vi "Build New Ballard MIL-STD-1553 Custom Device.vi"() -> ()   [LabVIEW 2020]
uses:
  <vilib>/addons/VeriStand Custom Device Scripting APIs/Ballard MIL-STD-1553/Shared/Address.ctl
  <vilib>/addons/VeriStand Custom Device Scripting APIs/Ballard MIL-STD-1553/Shared/Device Parameters.ctl
  <vilib>/addons/VeriStand Custom Device Scripting APIs/Ballard MIL-STD-1553/Shared/Initialization Method.ctl
  NationalInstruments.VeriStand.SystemDefinitionAPI
  AIM MIL-STD-1553 Scripting Example Support.lvlib
panel:
  in  "Example Documentation":string="Overview: Demonstrates using the Ballard MIL-STD-1553 scripting API to add and configure a new custom device from configuration data. \n\nInstructions:\n1. Specify the PXI Slot Number and Core Number for your Astronics MIL-STD-1553 hardware with Ballard technology.\n2. Specify the Hardware Configuration File. The hardware configuration file must be consistent with the schema installed by the Ballard hardware driver at \nC:\\Program Files (x86)\\Astronics Ballard Technology LabVIEW Driver\\Help\\index.html.\n3. (VeriStand) Optionally, to perform avionics bus communications with Ballard MIL-STD-1553 hardware you may:\n   a. Open the Ballard MIL-STD-1553 System Definition in VeriStand.\n   b. Configure the PXI Linux RT Target.\n   c. Deploy the scripted system definition."
  in  "Core Number":i32
  in  "PXI Slot Number":i32=2
  in  "Hardware Configuration File":path=path "Support/Ballard MIL-STD-1553 Hardware.xml"
  in  "Base System Definition File":path=path "Support/Base.nivssdf"
  in  "Output System Definition File":path=path "Support/Scripted Configuration Ballard MIL-STD-1553.nivssdf"
  out "Ballard MIL-STD-1553 System Definition":path
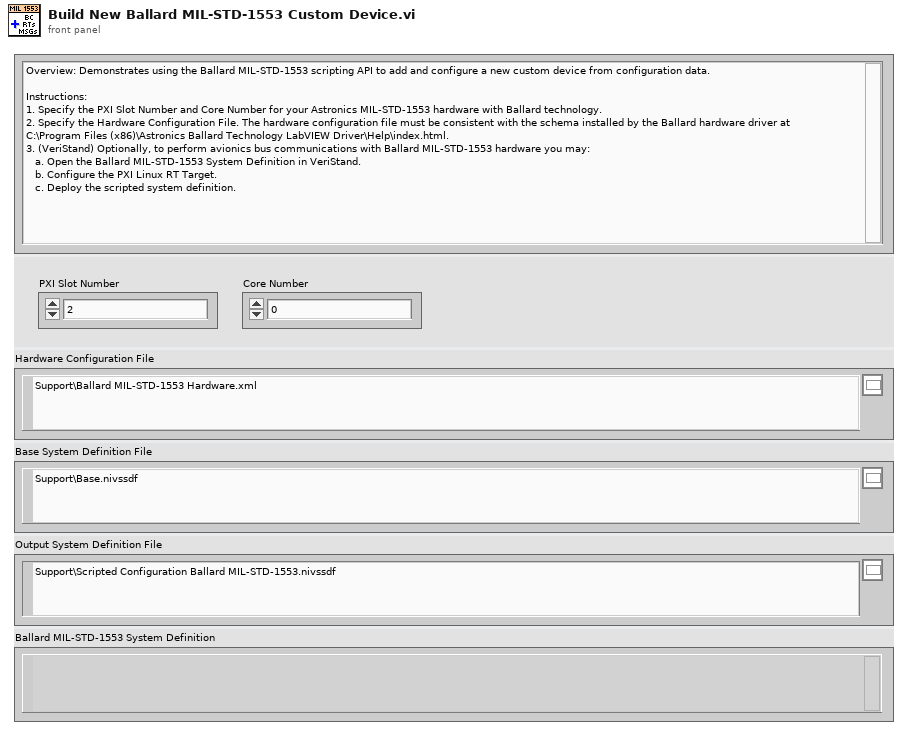
[diagram p1: front panel]
types:
  T1 = typedef "Device Parameters.ctl" = cluster{"initialization method":T2, "card number":i32, "PXI slot number":i32, "core number":i32}
  T2 = typedef "Initialization Method.ctl" = enum16{"PXI Slot Number", "Card Number"}
  T3 = typedef "Address.ctl" = u16
  T4 = cluster{"name":string, "message type":string, "Tx endpoint":cluster{"terminal address":u16, "subaddress":u16}, "Rx endpoint":cluster{"terminal address":u16, "subaddress":u16}, "create timestamp ch":bool, "mode code":u16, "number of words":u16, "parameters":cluster{"name":string, "default value":dbl, "unit":string, "parameter definition":cluster{"start index":i32, "size (bits)":i32, "encoding":enum16{"BNR", "BCD", "Discrete"}, "signed":bool, "multiplier":dbl, "offset":dbl}}[]}[]
  T5 = typedef "Custom Device API.lvlib/Custom Device Item Ref.ctl" = u64
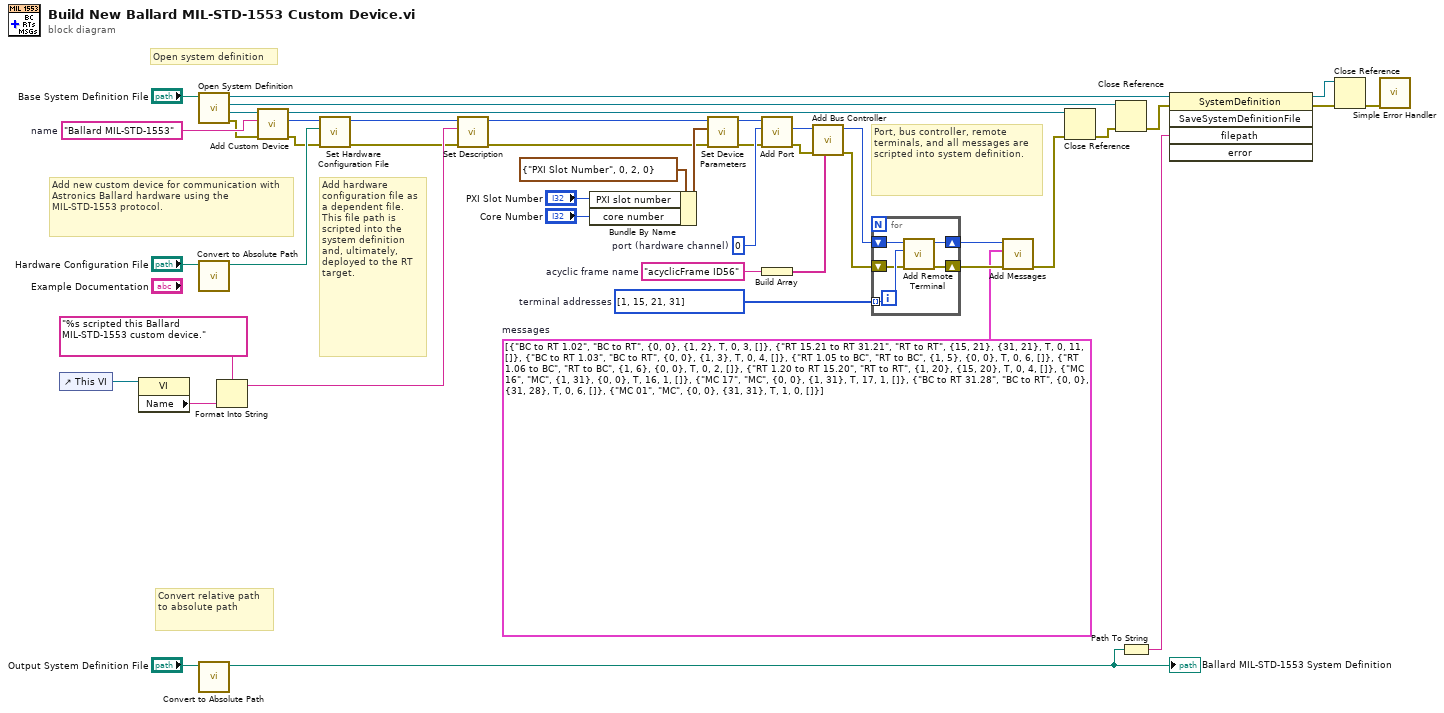
[diagram p0: block diagram]
diagram:
  w18 = T3[] [1, 15, 21, 31]  # terminal addresses
  w16 = "acyclicFrame ID56"  # acyclic frame name
  w12 = T4 [{"name"="BC to RT 1.02", "message type"="BC to RT", "Tx endpoint"={"terminal address"=0, "subaddress"=0}, "Rx endpoint"={"terminal address"=1, "subaddress"=2}, "create timestamp ch"=TRUE, "mode code"=0, "number of words"=3, "parameters"=[]}, {"name"="RT 15.21 to RT 31.21", "message type"="RT to RT", "Tx endpoint"={"terminal address"=15, "subaddress"=21}, "Rx endpoint"={"terminal address"=31, "subaddress"=21}, "create timestamp ch"=TRUE, "mode code"=0, "number of words"=11, "parameters"=[]}, {"name"="BC to RT 1.03", "message type"="BC to RT", "Tx endpoint"={"terminal address"=0, "subaddress"=0}, "Rx endpoint"={"terminal address"=1, "subaddress"=3}, "create timestamp ch"=TRUE, "mode code"=0, "number of words"=4, "parameters"=[]}, {"name"="RT 1.05 to BC", "message type"="RT to BC", "Tx endpoint"={"terminal address"=1, "subaddress"=5}, "Rx endpoint"={"terminal address"=0, "subaddress"=0}, "create timestamp ch"=TRUE, "mode code"=0, "number of words"=6, "parameters"=[]}, {"name"="RT 1.06 to BC", "message type"="RT to BC", "Tx endpoint"={"terminal address"=1, "subaddress"=6}, "Rx endpoint"={"terminal address"=0, "subaddress"=0}, "create timestamp ch"=TRUE, "mode code"=0, "number of words"=2, "parameters"=[]}, {"name"="RT 1.20 to RT 15.20", "message type"="RT to RT", "Tx endpoint"={"terminal address"=1, "subaddress"=20}, "Rx endpoint"={"terminal address"=15, "subaddress"=20}, "create timestamp ch"=TRUE, "mode code"=0, "number of words"=4, "parameters"=[]}, {"name"="MC 16", "message type"="MC", "Tx endpoint"={"terminal address"=1, "subaddress"=31}, "Rx endpoint"={"terminal address"=0, "subaddress"=0}, "create timestamp ch"=TRUE, "mode code"=16, "number of words"=1, "parameters"=[]}, {"name"="MC 17", "message type"="MC", "Tx endpoint"={"terminal address"=0, "subaddress"=0}, "Rx endpoint"={"terminal address"=1, "subaddress"=31}, "create timestamp ch"=TRUE, "mode code"=17, "number of words"=1, "parameters"=[]}, {"name"="BC to RT 31.28", "message type"="BC to RT", "Tx endpoint"={"terminal address"=0, "subaddress"=0}, "Rx endpoint"={"terminal address"=31, "subaddress"=28}, "create timestamp ch"=TRUE, "mode code"=0, "number of words"=6, "parameters"=[]}, {"name"="MC 01", "message type"="MC", "Tx endpoint"={"terminal address"=0, "subaddress"=0}, "Rx endpoint"={"terminal address"=31, "subaddress"=31}, "create timestamp ch"=TRUE, "mode code"=1, "number of words"=0, "parameters"=[]}]  # messages
  w24 = u16 0  # port (hardware channel)
  w33 = "Ballard MIL-STD-1553"  # name
  # "Add hardware configuration file as a dependent file. This file path is scripted into the system definition and, ultimately, deployed to the RT target."
  # "Port, bus controller, remote terminals, and all messages are scripted into system definition."
  # "Add new custom device for communication with Astronics Ballard hardware using the MIL-STD-1553 protocol."
  # "Convert relative path to absolute path"
  # "Open system definition"
  # "8."
  n1 = control-ref of="This VI"() -> (w27:refnum<vi>)
  n2 = property class="VI"(reference=w27) -> ("Name"=w26:string)  [unwired: 1 in, 2 out]
  n3 = call "Open System Definition.vi"("system definition file"="Base System Definition File") -> ("error out"=w29:errorcluster, "target"=w36:refnum<k24>, "root"=w31:refnum<k24>, "system definition"=w30:refnum<k24>)  [unwired: 7 in]
  n4 = call "Convert to Absolute Path.vi"("system definition file"="Hardware Configuration File") -> ("absolute path"=w35:path)  [unwired: 10 in]
  n5 = call "Convert to Absolute Path.vi"("system definition file"="Output System Definition File") -> ("absolute path"=w34:path)  [unwired: 10 in]
  "Ballard MIL-STD-1553 System Definition" <- w34
  n6 = Format Into String(format string="%s scripted this Ballard MIL-STD-1553 custom device." ("description"), w26) -> (resulting string=w25:string)  [unwired: 2 in, 1 out]
  n7 = call <vilib>:"Add Custom Device.vi"("error in"=w29, "name"=w33, "target in"=w36) -> ("error out"=w22:errorcluster, "Ballard MIL-STD 1553 custom device"=w23:T5, "target out"=w32:refnum<k24>)  [unwired: 6 in]
  n8 = call <vilib>:"Set Hardware Configuration File.vi"("error in"=w22, "hardware configuration file path"=w35, "Ballard MIL-STD 1553 custom device in"=w23) -> ("error out"=w10:errorcluster, "Ballard MIL-STD 1553 custom device out"=w11:T5)  [unwired: 7 in]
  n9 = call <vilib>:"Set Description.vi"("error in"=w10, "description"=w25, "Ballard MIL-STD 1553 custom device in"=w11) -> ("error out"=w3:errorcluster, "Ballard MIL-STD 1553 custom device out"=w8:T5)  [unwired: 7 in]
  n10 = Bundle By Name(cluster=T1 {"initialization method"=enum."PXI Slot Number", "card number"=0, "PXI slot number"=2, "core number"=0} ("device parameters"), "PXI slot number"="PXI Slot Number", "core number"="Core Number") -> (w5:T1)
  n11 = call <vilib>:"Set Device Parameters.vi"("error in"=w3, "device parameters"=w5, "Ballard MIL-STD 1553 custom device in"=w8) -> ("error out"=w4:errorcluster, "Ballard MIL-STD 1553 custom device out"=w7:T5)  [unwired: 7 in]
  n12 = call <vilib>:"Add Port.vi"("error in"=w4, "port number"=w24, "Ballard MIL-STD 1553 custom device in"=w7) -> ("error out"=w20:errorcluster, "port"=w21:T5)  [unwired: 6 in, 1 out]
  n13 = Build Array(w16) -> (w15:string[])
  n14 = call <vilib>:"Add Bus Controller.vi"("acyclic frame names"=w15, "error in"=w20, "port in"=w21) -> ("error out"=w17:errorcluster, "port out"=w19:T5)  [unwired: 6 in, 1 out]
  n15 = for {
    tunnel: w18 -> [w49] mode=indexing
    shift-right: [w47] -> w13
    shift-left: w17 -> [w48]
    shift-right: [w46] -> w14
    shift-left: w19 -> [w50]
    n16 = call <vilib>:"Add Remote Terminal.vi"("error in"=w48, "terminal address"=w49, "port in"=w50) -> ("error out"=w47:errorcluster, "port out"=w46:T5)  [unwired: 6 in, 1 out]
  }
  n17 = call <vilib>:"Add Messages.vi"("error in"=w13, "messages"=w12, "port in"=w14) -> ("error out"=w9:errorcluster)  [unwired: 7 in, 1 out]
  n18 = Close Reference(reference=w32, error in (no error)=w9) -> (error out=w38:errorcluster)
  n19 = Close Reference(reference=w31, error in (no error)=w38) -> (error out=w41:errorcluster)
  n20 = Path To String(path=w34) -> (string=w44:string)
  n21 = invoke class="SystemDefinition" method="SaveSystemDefinitionFile"(reference=w30, error in=w41, "filepath"=w44) -> (reference out=w42:refnum<k24>, error out=w43:errorcluster)  [unwired: 2 in, 3 out]
  n22 = Close Reference(reference=w42, error in (no error)=w43) -> (error out=w40:errorcluster)
  n23 = call <vilib>:"Simple Error Handler.vi"("error in (no error)"=w40) -> ()  [unwired: 1 in, 8 out]
